vi "FTW-Log-LookupMessenger.vi"(5 "Action":string, 7 "LoggerID":string, 11 "error in":errorcluster) -> (4 "Logger Messenger out":refnum<class "FTW-Messenger-Actor.lvclass">, 6 "Logged Event Broadcast":refnum<user-event>, 8 "Log Queue":refnum<queue>, 15 "error out":errorcluster)   [LabVIEW 2015]
uses:
  Messaging/Messenger.Actor/FTW-Messenger-Actor.lvclass
panel:
  # "Inputs"
  # "Outputs"
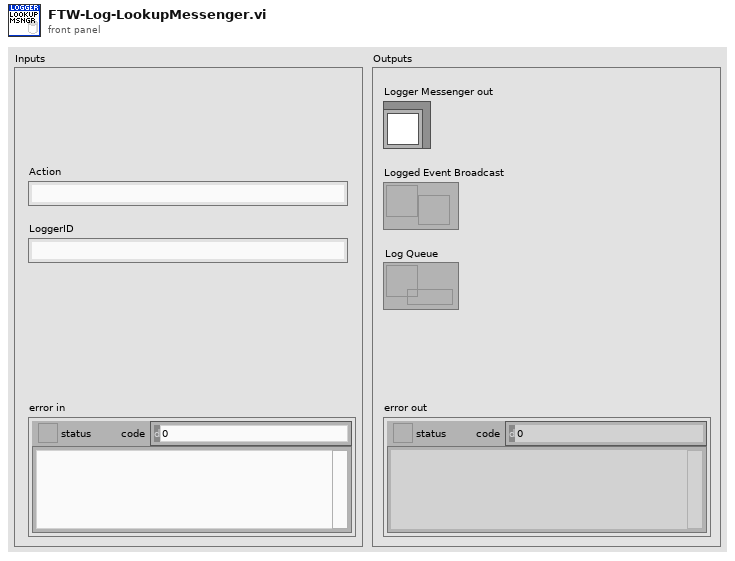
[diagram p1: front panel]
types:
  T1 = cluster{"Logger Messenger":refnum<class "FTW-Messenger-Actor.lvclass">, "Logged Event Broadcast":refnum<user-event>}
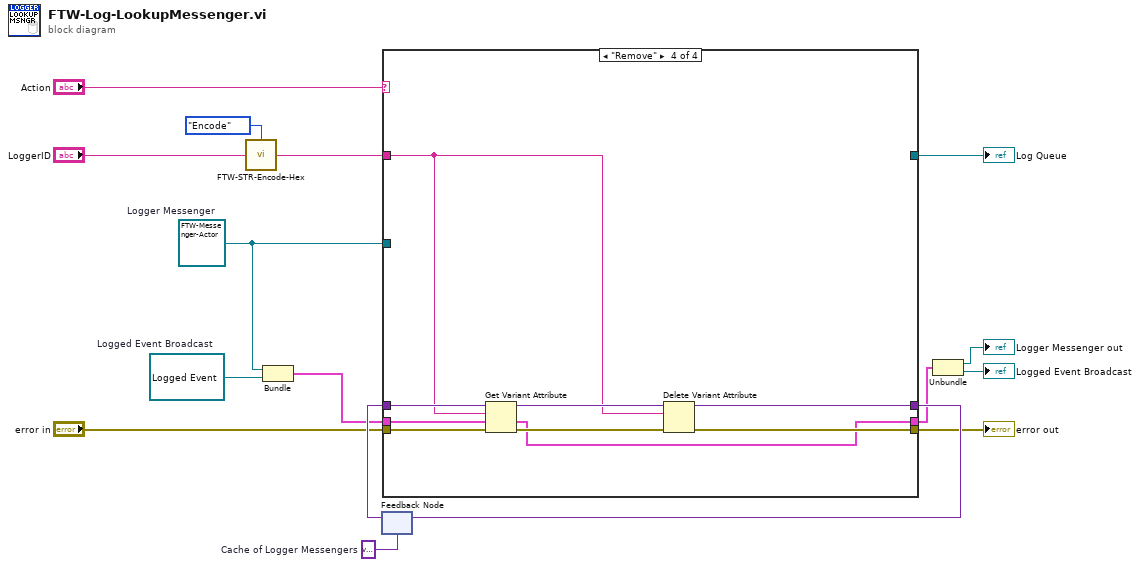
[diagram p0: block diagram]
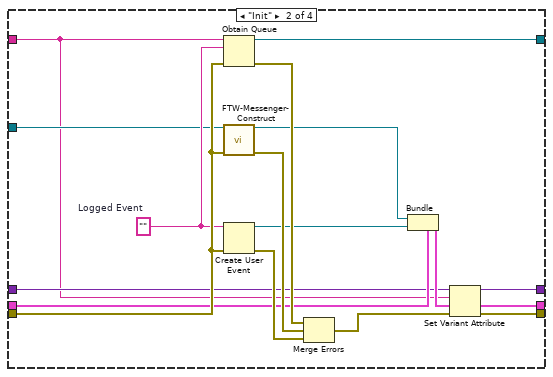
[diagram p3: hidden frame]
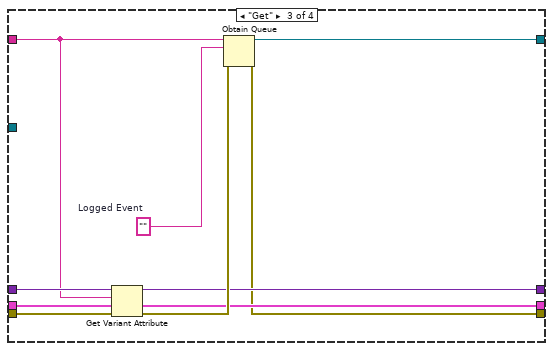
[diagram p4: hidden frame]
diagram:
  w6 = refnum<class "FTW-Messenger-Actor.lvclass"> refnum  # Logger Messenger
  w9 = refnum<user-event> refnum  # Logged Event Broadcast
  w16 = variant  # Cache of Logger Messengers
  n1 = call "FTW-STR-Encode-Hex.vi"("Input"="LoggerID", "Direction"=enum16{"Encode", "Decode"}."Encode") -> ("Output"=w7:string)
  n2 = Bundle("Logger Messenger"=w6, "Logged Event Broadcast"=w9) -> (w10:T1)  [unwired: 1 in]
  n3 = feedback #1(w16) -> (w15:variant)
  n4 = case shown="\"Remove\"" "Action" {
    tunnel: w15 -> [w19 w23 w44 w54]
    tunnel: [w19 w31 w37 w53] -> w14
    tunnel: "error in" -> [w17 w34 w43 w52]
    tunnel: w10 -> [w18 w24 w41 w51]
    tunnel: [w17 w29 w36 w50] -> w8
    tunnel: w7 -> [_ w22 w40 w47]
    tunnel: w6 -> [_ w28 _ _]
    tunnel: [w18 w27 w38 w46] -> w3
    tunnel: [_ w21 w39 _] -> w2
    frame Default {
    }
    frame "Init" {
      w30 = ""  # Logged Event
      n5 = Obtain Queue(name (unnamed)=w22, element data type=w30, error in (no error)=w34) -> (queue out=w21:refnum<queue>, error out=w32:errorcluster)  [unwired: 2 in, 1 out]
      n6 = call-dynamic "FTW-Messenger-Construct.vi"("Messenger Type"=w28, "error in"=w34) -> ("Actor Messenger"=w25:refnum<class "FTW-Messenger-Actor.lvclass">, "error out"=w33:errorcluster)  [unwired: 12 in]
      n7 = Create User Event(user event datatype=w30, error in=w34) -> (user event=w20:refnum<user-event>, error out=w35:errorcluster)
      n8 = Merge Errors(w32, w33, w35) -> (w26:errorcluster)
      n9 = Bundle(cluster=w24, "Logger Messenger"=w25, "Logged Event Broadcast"=w20) -> (w27:T1)
      n10 = Set Variant Attribute(Variant=w23, name=w22, value=w27, error in=w26) -> (Variant out=w31:variant, error out=w29:errorcluster)  [unwired: 1 out]
    }
    frame "Get" {
      w42 = ""  # Logged Event
      n11 = Get Variant Attribute(Variant=w44, name=w40, default value (empty Variant)=w41, error in=w43) -> (duplicate Variant=w37:variant, value=w38:T1, error out=w45:errorcluster)  [unwired: 1 out]
      n12 = Obtain Queue(name (unnamed)=w40, element data type=w42, error in (no error)=w45) -> (queue out=w39:refnum<queue>, error out=w36:errorcluster)  [unwired: 2 in, 1 out]
    }
    frame "Remove" {
      n13 = Get Variant Attribute(Variant=w54, name=w47, default value (empty Variant)=w51, error in=w52) -> (duplicate Variant=w48:variant, value=w46:T1, error out=w49:errorcluster)  [unwired: 1 out]
      n14 = Delete Variant Attribute(4:w49, 6:w47, 7:w48) -> (0:w50:errorcluster, 3:w53:variant)  [unwired: 1 out]
    }
  }
  "error out" <- w8
  "Log Queue" <- w2
  n15 = feedback-in #1(w14) -> ()
  n16 = Unbundle(w3) -> ("Logger Messenger"=→"Logger Messenger out":refnum<class "FTW-Messenger-Actor.lvclass">, "Logged Event Broadcast"=→"Logged Event Broadcast":refnum<user-event>)
